vi "cobat.vi"() -> ()   [LabVIEW 2015, in "Untitled Library 3.lvlib"]
uses:
  Untitled Library 3.lvlib
  <vilib>/rvi/Emulation/niFpgaGetClockAttributes.vi
  <vilib>/rvi/Emulation/niFpgaSctlEmulationGetInTimedLoop.vi
  <vilib>/rvi/Emulation/niFpgaEmulationReportErrorSimple.vi
  <vilib>/rvi/eio/common/nirviEmuTemplateMethod_errors.vi
  <vilib>/rvi/Emulation/niFpgaCriticalErrorInLSC.vi
  <vilib>/eio/EIONode/EIONode.xnode
panel:
  in  "STOP":bool
  in  "x":u16
  in  "y":u16
  out "FPGA I/O Out":refnum<k21>
  out "LED":bool
  in  "Count(Ticks)":u32
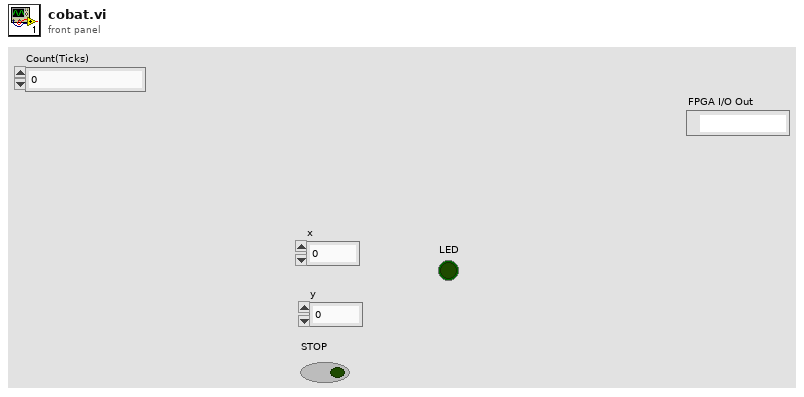
[diagram p1: front panel]
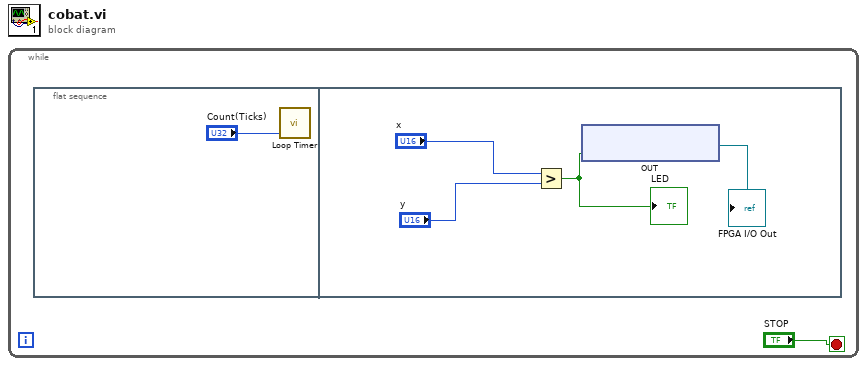
[diagram p0: block diagram]
diagram:
  n1 = while {
    stop <- "STOP" stop-if-true
    n2 = flat-sequence {
      frame #0 {
        n3 = call "Loop Timer"("Count(Ticks)"="Count(Ticks)") -> ()  [unwired: 1 out]
      }
      frame #1 {
        n4 = Greater?(x="x", y="y") -> (0:w5:bool)
        "LED" <- w5
        n5 = xnode "OUT"("ConnectorB/DIO4"=w5) -> ("FPGA I/O Out"=→"FPGA I/O Out":refnum<k21>)  [unwired: 1 in]
      }
    }
  }
